vi "Get String.vi"(0 "Session Handle in":T1, 5 "CMD":string="R1", 11 "error in":errorcluster) -> (4 "Session Handle out":T1, 6 "DataOut":string, 15 "error out":errorcluster)   [LabVIEW 2014, in "Serial Session.lvclass"]
doc: "Retrieve a string from the port - no conversion required."
uses:
  Serial Session.lvclass
  Typedefs/Session Handle.ctl
  Asynchronous Read.vi
  Asynchronous Write.vi
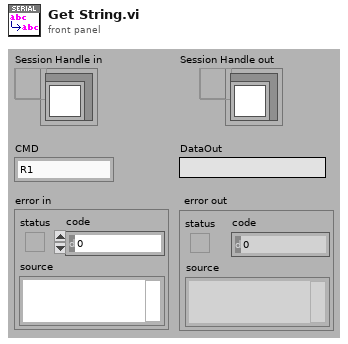
[diagram p1: front panel]
types:
  T1 = typedef "Serial Session.lvclass/Session Handle.ctl" = refnum<data-value>
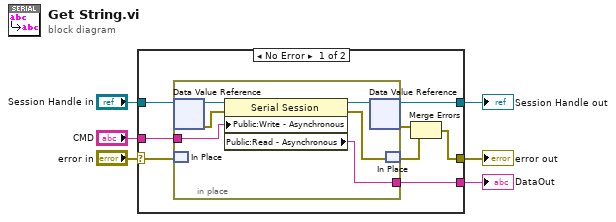
[diagram p0: block diagram]
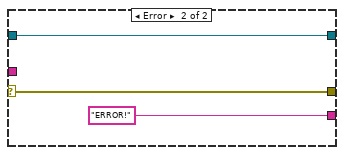
[diagram p2: hidden frame]
diagram:
  n1 = case shown="No Error" "error in" {
    selector: "error in" -> [w9 w22]
    tunnel: "Session Handle in" -> [w14 w23]
    tunnel: [w13 w23] -> w5
    tunnel: [w10 w22] -> w4
    tunnel: "CMD" -> [w8 _]
    tunnel: [w7 "ERROR!"] -> w1
    frame No Error {
      n2 = in-place {
        in-place-border: w8 -> [w16]
        in-place-border: [w15] -> w7
        n3 = in-place-dvr #1(w14) -> (w18:refnum<class "Serial Session.lvclass">, w19:errorcluster)
        n4 = in-place-match #2(w9) -> ()  [unwired: 1 out]
        n5 = property class="Serial Session"(reference=w18, error in=w19, "Public:Write - Asynchronous"=w16) -> (reference out=w17:refnum<class "Serial Session.lvclass">, error out=w20:errorcluster, "Public:Read - Asynchronous"=w15:string)
        n6 = in-place-dvr #1(w17) -> (w13:T1, w11:errorcluster)
        n7 = in-place-match #2(w20) -> (w12:errorcluster)
      }
      n8 = Merge Errors(w11, w12) -> (w10:errorcluster)
    }
    frame Error {
    }
  }
  "Session Handle out" <- w5
  "error out" <- w4
  "DataOut" <- w1
